vi "ConvertCommandArgumentsToUnsigned16.vi"(11 "Command":T1) -> (3 "Numérique":u16)   [LabVIEW 2021]
uses:
  CommandType.ctl
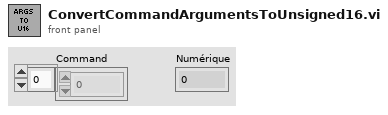
[diagram p1: front panel]
types:
  T1 = typedef "CommandType.ctl" = u8[]
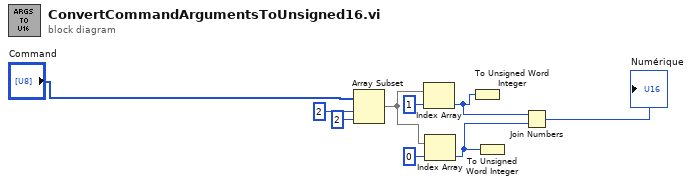
[diagram p0: block diagram]
diagram:
  n1 = Array Subset(array="Command", index=2 ("indice"), length=2 ("longueur")) -> (w5:T1)
  n2 = Index Array(array=w5, index=1 ("indice")) -> (element=w6:u8)
  n3 = Index Array(array=w5, index=0 ("indice")) -> (element=w7:u8)
  n4 = To Unsigned Word Integer(number=w6) -> ()  [unwired: 1 out]
  n5 = To Unsigned Word Integer(number=w7) -> ()  [unwired: 1 out]
  n6 = Join Numbers(hi=w6, lo=w7) -> ((hi.lo)=→"Numérique":u16)
